vi "Configure Channels.vi"(8 "error in":errorcluster, 11 "Scope PXI Base CFG in":refnum<class "Scope PXI Base CFG.lvclass">) -> (0 "error out":errorcluster, 3 "Scope PXI Base CFG out":refnum<class "Scope PXI Base CFG.lvclass">)   [LabVIEW 2023, in "Scope PXI Base CFG.lvclass"]
uses:
  Scope PXI Base CFG.lvclass
  <instrlib>/niScope/Controls/niScope vertical coupling.ctl
  Configuration/Configuration JSON/Configuration JSON Base/CFG JSON.lvclass/CFG JSON.ctl
  Scope PXI Base CFG.lvclass/Scope PXI Base CFG.ctl
  7cfe5669-d9a9-4cf8-b296-982c00835eb7.vi
  <vilib>/JDP Science/JSONtext/Find Item.vi
  <vilib>/JDP Science/JSONtext/Next JSON Value.vi
  <vilib>/JDP Science/JSONtext/String Subset.vi
  <vilib>/JDP Science/JSONtext/Parsing/Advance past next JSON Value (inlined COPY).vi
  <vilib>/JDP Science/JSONtext/Parsing/Advance past whitespace.vi
  <vilib>/JDP Science/JSONtext/Parsing/Advance past String.vi
  <vilib>/JDP Science/JSONtext/Parsing/Advance past Number.vi
  <vilib>/JDP Science/JSONtext/Parsing/Advance past Line Ending.vi
  <vilib>/JDP Science/JSONtext/Parsing/Parse Full Path or Item Name.vi
  <vilib>/JDP Science/JSONtext/Parsing/Advance past Array.vi
  <vilib>/JDP Science/JSONtext/Parsing/Advance past Object.vi
  <vilib>/JDP Science/JSONtext/support/Error Cluster From Code.vi
  <vilib>/JDP Science/JSONtext/Offset/Find Item Locations by Path.vi
  <vilib>/JDP Science/JSONtext/JSON text to Variant.vi
  <vilib>/Utility/error.llb/Error Cluster From Error Code.vi
  <vilib>/JDP Science/JSONtext/LVClass Serializer/JSONtext LVClass Serializer.lvclass
  <vilib>/ErrorRing/Error Ring.xnode
  Configuration/Configuration JSON/Configuration JSON Base/CFG JSON.lvclass
panel:
  out "input impedance":u32(ring)=2 items=["1 mega ohm"=0, "50 ohms"=2]
  out "vertical coupling":T1=1 caption="vertical coupling (DC)" items=["AC", "DC", "Ground"]
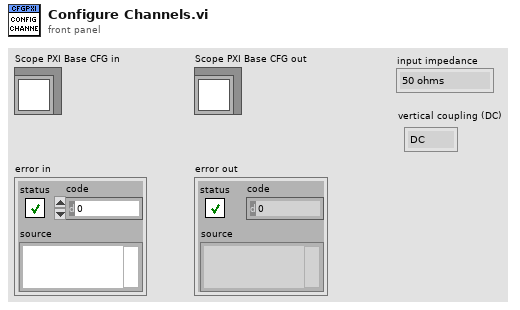
[diagram p1: front panel]
types:
  T1 = typedef "niScope vertical coupling.ctl" = i32
  T2 = cluster{"Enabled":bool, "Impedance":string, "Max Frequency":dbl, "Vertical Coupling":string, "Probe Attenuation":dbl, "Name":string, "Vertical Range":dbl, "Vertical Offset":dbl}[]
  T3 = typedef "LVStringsAndValuesArrayTypeDef_U32.ctl" = cluster{"String":string, "Value":u32}[]
  T4 = typedef "LVStringsAndValuesArrayTypeDef_I32.ctl" = cluster{"String":string, "Value":i32}[]
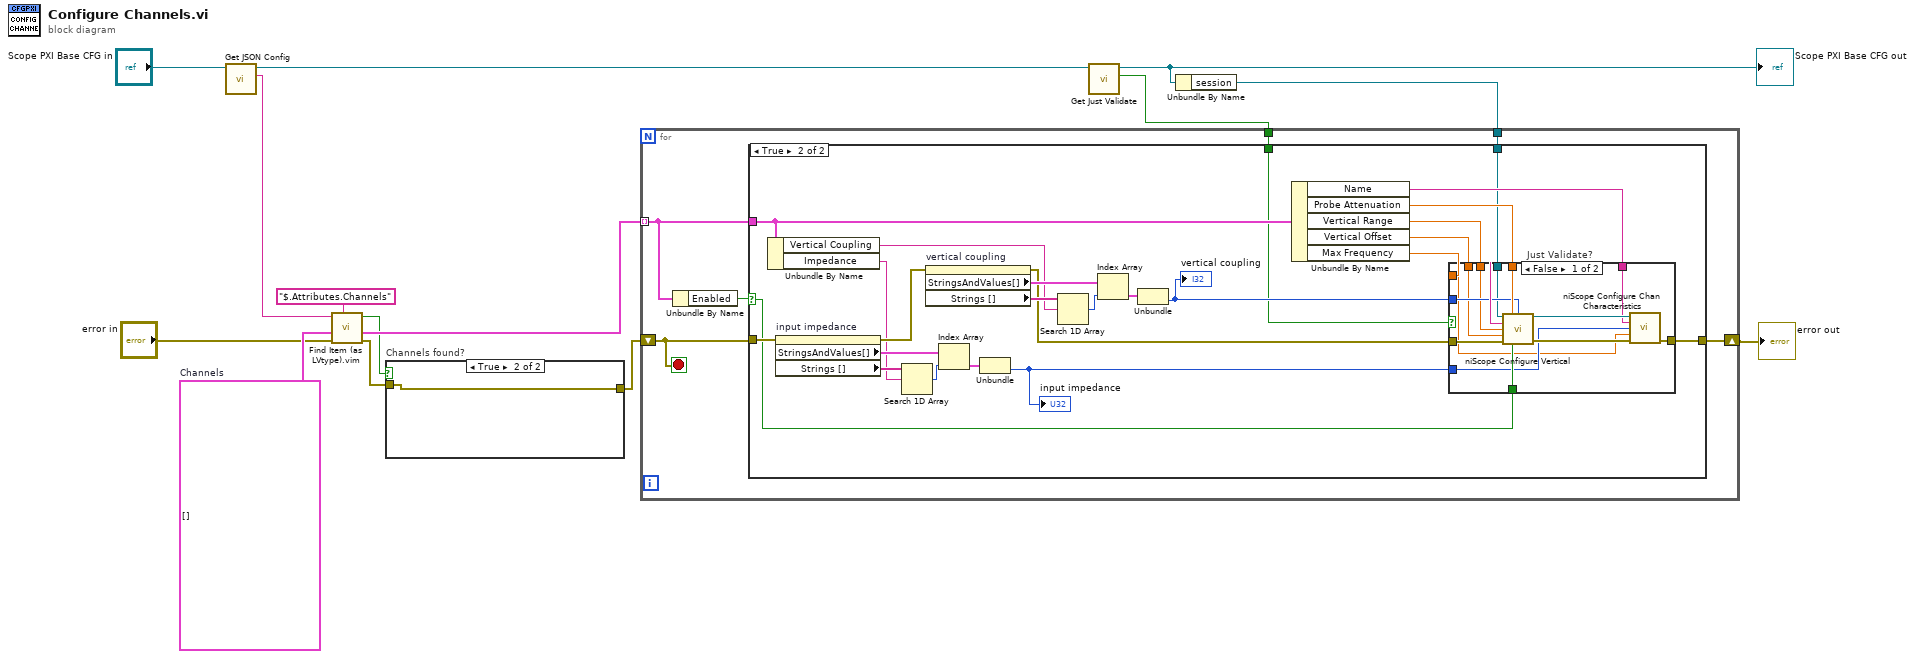
[diagram p0: block diagram]
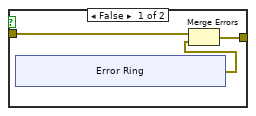
[diagram p2: hidden frame]
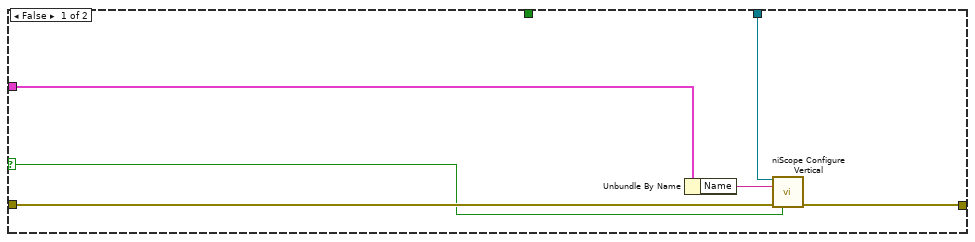
[diagram p3: hidden frame]
diagram:
  w9 = T2 []  # Channels
  n1 = call "Get JSON Config.vi"("CFG Base in"="Scope PXI Base CFG in") -> ("<JSON>Config>"=w11:string, "CFG Base out"=w5:refnum<class "Scope PXI Base CFG.lvclass">)  [unwired: 9 in]
  n2 = call "Find Item (as LVtype).vim"("$Path or Item Name"="$.Attributes.Channels", "error in (no error)"="error in", "Data Type and Default Value"=w9, "JSON"=w11) -> ("error out"=w6:errorcluster, "Data"=w13:T2, "Found"=w7:bool)  [unwired: 4 in, 1 out]
  n3 = case "Channels found?" shown="True" w7 {
    tunnel: [w17 w23] -> w8
    tunnel: w6 -> [w15 w23]
    frame False {
      n4 = xnode "Error Ring"() -> ("error out"=w16:errorcluster)
      n5 = Merge Errors(w15, w16) -> (w17:errorcluster)
    }
    frame True {
    }
  }
  n6 = call "Get Just Validate.vi"("CFG JSON Base in"=w5) -> ("Just Validate"=w2:bool, "CFG JSON Base out"=w3:refnum<class "Scope PXI Base CFG.lvclass">)  [unwired: 9 in]
  "Scope PXI Base CFG out" <- w3
  n7 = Unbundle By Name(w3) -> ("session"=w4:refnum<k15>)
  n8 = for {
    shift-right: [w29] -> w10
    shift-left: w8 -> [w26]
    tunnel: w13 -> [w28] mode=indexing
    tunnel: w4 -> [w25]
    tunnel: w2 -> [w24]
    stop <- w26 stop-if-true
    n9 = Unbundle By Name(w28) -> ("Enabled"=w27:bool)
    n10 = case shown="True" w27 {
      selector: w27 -> [w33 w46]
      tunnel: [w35 w60] -> w29
      tunnel: w26 -> [w34 w51]
      tunnel: w28 -> [w32 w47]
      tunnel: w25 -> [w31 w37]
      tunnel: w24 -> [_ w36]
      frame False {
        n11 = Unbundle By Name(w32) -> ("Name"=w30:string)
        n12 = call <instrlib>:"niScope Configure Vertical.vi"("instrument handle"=w31, "channels"=w30, "error in"=w34, "channel enabled"=w33) -> ("error out"=w35:errorcluster)  [unwired: 10 in, 1 out]
      }
      frame True {
        n13 = Unbundle By Name(w47) -> ("Vertical Coupling"=w48:string, "Impedance"=w49:string)
        n14 = property on="input impedance" class="Ring (strict)"(error in=w51) -> (error out=w50:errorcluster, "StringsAndValues[]"=w57:T3, "Strings []"=w56:string[])  [unwired: 1 in, 1 out]
        n15 = Search 1D Array(1D array=w56, element=w49) -> (index of element=w58:i32)  [unwired: 1 in]
        n16 = property on="vertical coupling" class="Ring (strict)"(error in=w50) -> (error out=w40:errorcluster, "StringsAndValues[]"=w53:T4, "Strings []"=w55:string[])  [unwired: 1 in, 1 out]
        n17 = Index Array(array=w57, index=w58) -> (element=w59:cluster{"String":string, "Value":u32})
        n18 = Unbundle(w59) -> ("Value"=w39:u32)  [unwired: 1 out]
        "input impedance" <- w39
        n19 = Search 1D Array(1D array=w55, element=w48) -> (index of element=w54:i32)  [unwired: 1 in]
        n20 = Index Array(array=w53, index=w54) -> (element=w52:cluster{"String":string, "Value":i32})
        n21 = Unbundle(w52) -> ("Value"=w43:i32)  [unwired: 1 out]
        "vertical coupling" <- w43
        n22 = Unbundle By Name(w47) -> ("Name"=w45:string, "Probe Attenuation"=w44:dbl, "Vertical Range"=w42:dbl, "Vertical Offset"=w41:dbl, "Max Frequency"=w38:dbl)
        n23 = case "Just Validate?" shown="False" w36 {
          tunnel: [w73 w74] -> w60
          tunnel: w46 -> [w70 _]
          tunnel: w45 -> [w69 _]
          tunnel: w44 -> [w68 _]
          tunnel: w43 -> [w67 _]
          tunnel: w42 -> [w66 _]
          tunnel: w41 -> [w65 _]
          tunnel: w40 -> [w64 w74]
          tunnel: w39 -> [w63 _]
          tunnel: w38 -> [w62 _]
          tunnel: w37 -> [w61 _]
          frame False {
            n24 = call <instrlib>:"niScope Configure Vertical.vi"("instrument handle"=w61, "probe attenuation"=w68, "vertical coupling"=w67, "channels"=w69, "vertical range"=w66, "vertical offset"=w65, "error in"=w64, "channel enabled"=w70) -> ("instrument handle out"=w71:refnum<k15>, "error out"=w72:errorcluster)  [unwired: 6 in]
            n25 = call <instrlib>:"niScope Configure Chan Characteristics.vi"("instrument handle"=w71, "channels"=w69, "input impedance"=w63, "maximum input frequency"=w62, "error in"=w72) -> ("error out"=w73:errorcluster)  [unwired: 9 in, 1 out]
          }
          frame True {
          }
        }
      }
    }
  }
  "error out" <- w10
